vi "averaged_ilemt_data.vi"(8 "error in":errorcluster, 9 "Position":dbl[](array[numeric]) format="%#_3p", 10 "Point time (ms)":u32=1, 11 "Settling time (ms)":u32=1) -> (0 "error out":errorcluster, 1 "End timestamp":T1, 2 "Start timestamp":T1, 3 "Result string":string)   [LabVIEW 2024]
uses:
  system/relative_and_absolute_ts.ctl
  <vilib>/Utility/error.llb/Trim Whitespace One-Sided.vi
  main/ilemt_globals.vi
panel:
  # "Get ILEMT calibration log text output record, averaging over specified time. A queue read error such as timeout will terminate, leaving the output undefined."
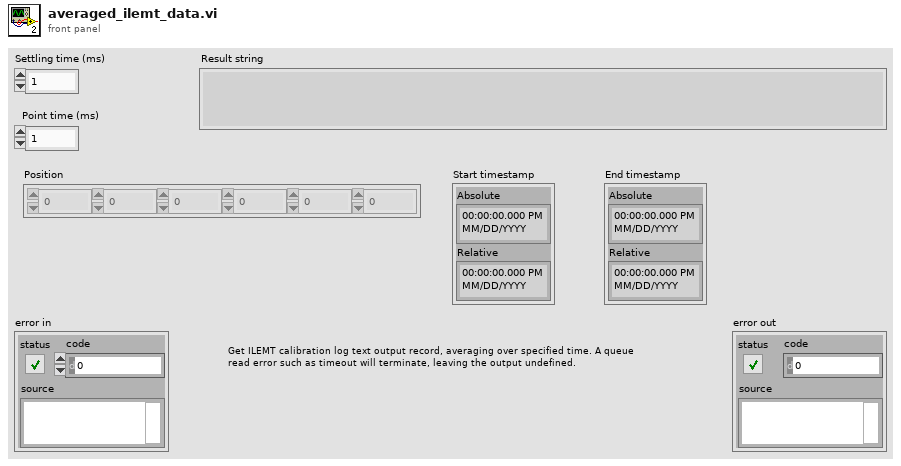
[diagram p1: front panel]
types:
  T1 = typedef "relative_and_absolute_ts.ctl" = cluster{"Absolute":timestamp, "Relative":timestamp}
  T2 = typedef "modulation_info.ctl" = cluster{"Fs full":dbl, "Fs high":dbl, "Fs low":dbl, "Read size":i32, "FFT size low":i32, "df low":dbl, "High carriers":dbl[], "Low carriers":dbl[], "Hi channels at low":i32[]}
  T3 = cluster{"seconds since 1Jan1904":timestamp, timestamp}
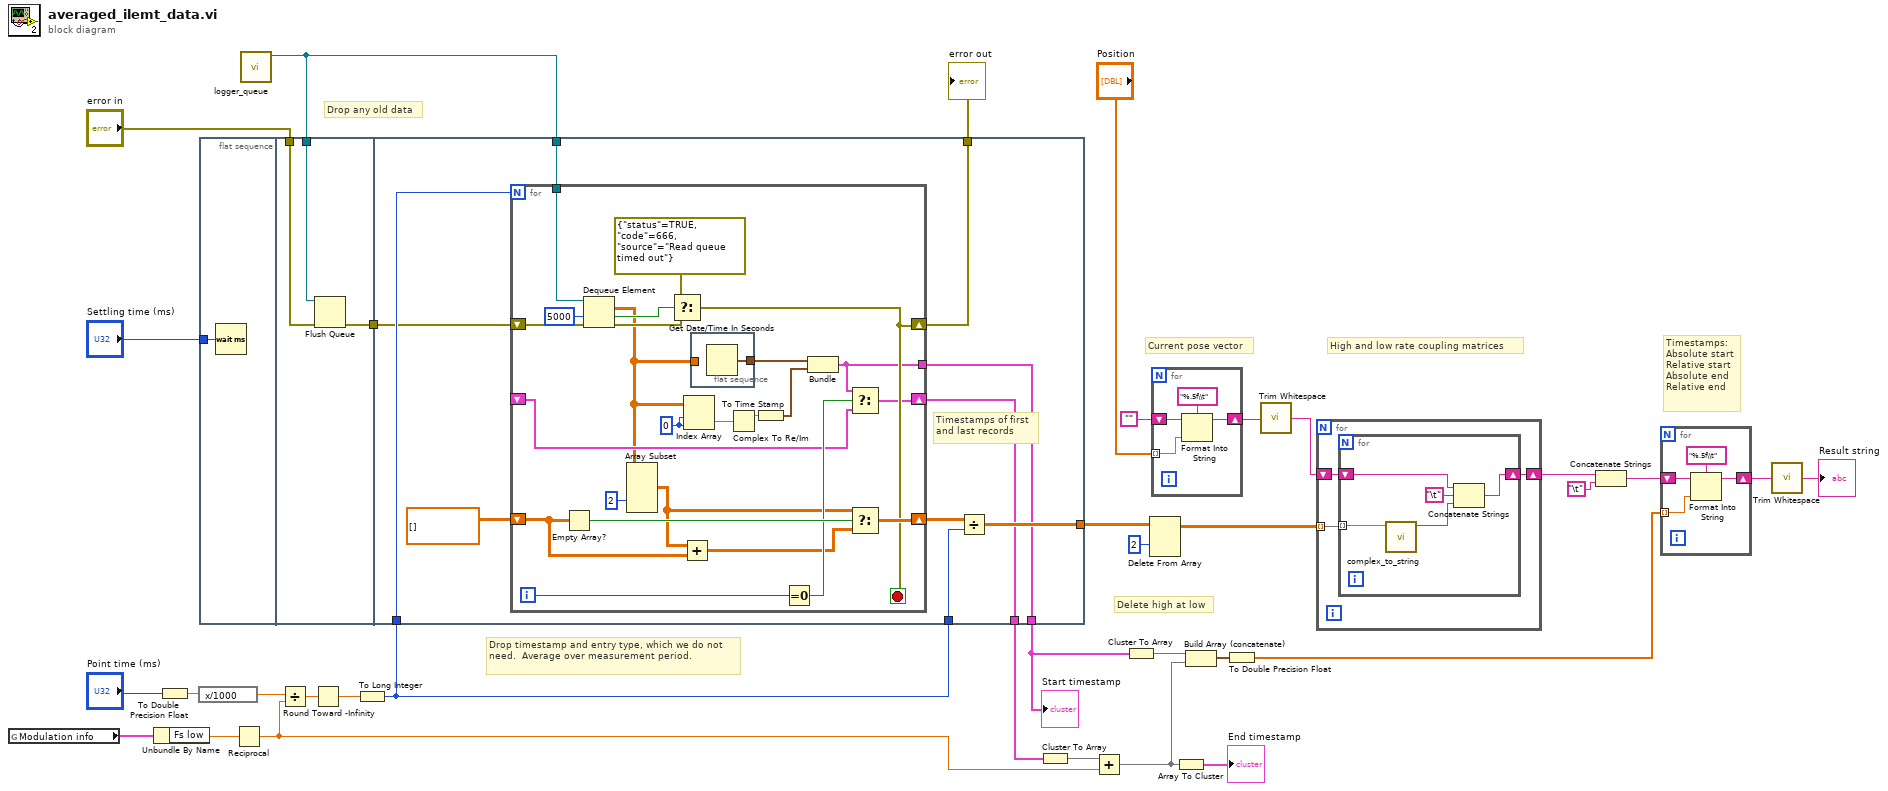
[diagram p0: block diagram]
diagram:
  # "Timestamps:\nAbsolute start\nRelative start\nAbsolute end\nRelative end"
  # "Current pose vector"
  # "High and low rate coupling matrices"
  # "Delete high at low"
  # "Drop any old data"
  # "Drop timestamp and entry type, which we do not need.  Average over measurement period."
  n1 = global read "ilemt_globals.vi" "Modulation info"() -> (w33:T2)
  n2 = Unbundle By Name(w33) -> ("Fs low"=w32:dbl)
  n3 = To Double Precision Float(number="Point time (ms)") -> (double precision float=w31:dbl)
  n4 = expression code="x/1000"(w31) -> (w29:dbl)
  n5 = flat-sequence {
    tunnel: "Settling time (ms)" -> [w35]
    tunnel: w26 -> [w38]
    tunnel: "error in" -> [w37]
    tunnel: [w36] -> w24
    tunnel: w25 -> [w48]
    tunnel: w26 -> [w47]
    tunnel: w25 -> [w44]
    tunnel: w24 -> [w43]
    tunnel: [w42] -> w23
    tunnel: [w41] -> w16
    tunnel: [w40] -> w14
    tunnel: [w39] -> w10
    frame #0 {
      n6 = Wait (ms)(milliseconds to wait=w35) -> ()  [unwired: 1 out]
    }
    frame #1 {
      n7 = Flush Queue(queue=w38, error in (no error)=w37) -> (error out=w36:errorcluster)  [unwired: 2 out]
    }
    frame #2 {
      # "Timestamps of first and last records"
      n8 = for {
        N: w48 -> [_]
        tunnel: w47 -> [w71]
        shift-right: [w68] -> w45
        shift-left: cdb[][] [] -> [w67]
        shift-right: [w61] -> w42
        shift-left: w43 -> [w70]
        tunnel: [w56] -> w39
        shift-right: [w57] -> w40
        shift-left: _ -> [w58]
        i -> [w72]
        stop <- w61 stop-if-true
        w60 = 0 ("disabled index (col)")
        n9 = Empty Array?(array=w67) -> (empty?=w69:bool)
        n10 = Dequeue Element(queue=w71, timeout in ms (-1)=5000, error in (no error)=w70) -> (element=w51:cdb[][], timed out?=w64:bool, error out=w63:errorcluster)  [unwired: 1 out]
        n11 = Array Subset(array=w51, index (col)=2 ("index")) -> (w52:cdb[][])  [unwired: 3 in]
        n12 = Select(t=errorcluster {"status"=TRUE, "code"=666, "source"="Read queue timed out"} ("error out"), s=w64, f=w63) -> (s? t:f=w61:errorcluster)
        n13 = Add(x=w52, y=w67) -> (x+y=w53:cdb[][])
        n14 = Index Array(array=w51, index (row)=w60, index (col)=w60) -> (element=w55:cdb)
        n15 = flat-sequence {
          tunnel: [w73] -> w50
          tunnel: w51 -> [_]
          frame #0 {
            n16 = Get Date/Time In Seconds() -> (seconds since 1Jan1904=w73:timestamp)
          }
        }
        n17 = Complex To Re/Im(x + iy=w55) -> (x=w54:dbl)  [unwired: 1 out]
        n18 = To Time Stamp(1:w54) -> (0:w49:timestamp)
        n19 = Equal To 0?(x=w72) -> (x = 0?=w59:bool)
        n20 = Bundle("seconds since 1Jan1904"=w50, w49) -> (w56:T3)  [unwired: 1 in]
        n21 = Select(t=w56, s=w59, f=w58) -> (s? t:f=w57:T3)
        n22 = Select(t=w52, s=w69, f=w53) -> (s? t:f=w68:cdb[][])
      }
      n23 = Divide(x=w45, y=w44) -> (x/y=w41:cdb[][])
    }
  }
  n24 = Reciprocal(x=w32) -> (1/x=w12:dbl)
  n25 = call "logger_queue.vi"() -> ("queue out"=w26:refnum<queue>)  [unwired: 10 in, 1 out]
  n26 = Divide(x=w29, y=w12) -> (x/y=w28:dbl)
  n27 = Round Toward -Infinity(1:w28) -> (0:w15:dbl)
  n28 = To Long Integer(number=w15) -> (32bit integer=w25:i32)
  n29 = Cluster To Array(cluster=w14) -> (array=w13:timestamp[])
  n30 = Add(x=w13, y=w12) -> (x+y=w8:timestamp[])
  n31 = Cluster To Array(cluster=w10) -> (array=w9:timestamp[])
  n32 = Delete From Array(array=w16, index (row)=2) -> (array with subset deleted=w21:cdb[][])  [unwired: 2 in, 1 out]
  n33 = for {
    tunnel: "Position" -> [w74] mode=indexing
    shift-right: [w75] -> w18
    shift-left: "" -> [w76]
    n34 = Format Into String(format string="%.5f\\t" ("format (%.3f)"), initial string=w76, w74) -> (resulting string=w75:string)  [unwired: 1 in, 1 out]
  }
  n35 = Array To Cluster(array=w8) -> (cluster=→"End timestamp":cluster{"[0]":timestamp, "[1]":timestamp})
  n36 = Build Array (concatenate)(w9, w8) -> (w7:timestamp[])
  n37 = To Double Precision Float(number=w7) -> (double precision float=w6:dbl[])
  n38 = call <vilib>:"Trim Whitespace.vi"("string"=w18) -> ("trimmed string"=w17:string)  [unwired: 1 in]
  n39 = for {
    tunnel: w21 -> [w80] mode=indexing
    shift-right: [w78] -> w3
    shift-left: w17 -> [w79]
    n40 = for {
      tunnel: w80 -> [w85] mode=indexing
      shift-right: [w81] -> w78
      shift-left: w79 -> [w82]
      n41 = call "complex_to_string.vi"("Numeric"=w85) -> ("output string"=w84:string)  [unwired: 10 in]
      n42 = Concatenate Strings(w82, "\t" ("string"), w84) -> (w81:string)
    }
  }
  n43 = Concatenate Strings(w3, "\t" ("string")) -> (w1:string)
  n44 = for {
    tunnel: w6 -> [w86] mode=indexing
    shift-right: [w87] -> w5
    shift-left: w1 -> [w88]
    n45 = Format Into String(format string="%.5f\\t" ("format (%.3f)"), initial string=w88, w86) -> (resulting string=w87:string)  [unwired: 1 in, 1 out]
  }
  n46 = call <vilib>:"Trim Whitespace.vi"("string"=w5) -> ("trimmed string"=→"Result string":string)  [unwired: 1 in]
  "error out" <- w23
  "Start timestamp" <- w10
